vi "Configure Data Logging.vi"(7 "State (False)":bool, 8 "error in (no error)":errorcluster, 9 "Duration (30 minutes)":i32=30, 10 "Source (0:Channel 1)":i32(ring) items=["Channel 1", "Channel 2", "Channel 3", "Channel 4", "Math", "FFT"], 11 "VISA resource name":refnum<visa-resource-name>) -> (0 "error out":errorcluster, 3 "VISA resource name out":refnum<visa-resource-name>)   [LabVIEW 2015, in "Tektronix TDS 200 1000 2000 Series.lvlib"]
doc: "This VI configures the settings for the data logging."
uses:
  <instrlib>/Tektronix TDS 200 1000 2000 Series/Tektronix TDS 200 1000 2000 Series.lvlib
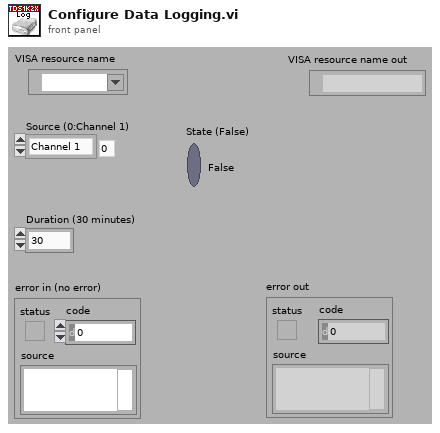
[diagram p1: front panel]
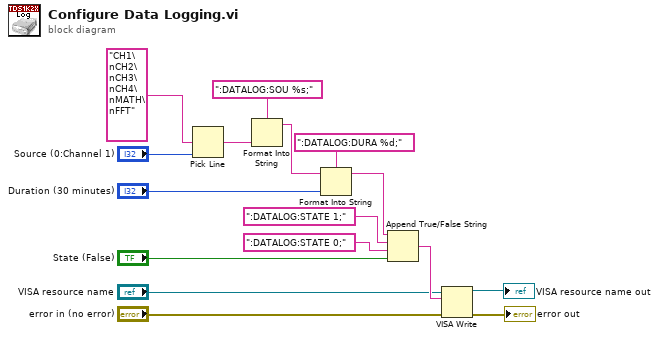
[diagram p0: block diagram]
diagram:
  n1 = Pick Line(multi-line string="CH1\nCH2\nCH3\nCH4\nMATH\nFFT", line index="Source (0:Channel 1)") -> (output string=w11:string)  [unwired: 1 out]
  n2 = Format Into String(format string=":DATALOG:SOU %s;", w11) -> (resulting string=w8:string)  [unwired: 2 in, 1 out]
  n3 = Format Into String(format string=":DATALOG:DURA %d;", initial string=w8, "Duration (30 minutes)") -> (resulting string=w7:string)  [unwired: 1 in, 1 out]
  n4 = Append True/False String(1:"State (False)", 2:":DATALOG:STATE 0;", 3:":DATALOG:STATE 1;", 4:w7) -> (0:w9:string)
  n5 = VISA Write(VISA resource name="VISA resource name", write buffer=w9, error in (no error)="error in (no error)") -> (VISA resource name out=→"VISA resource name out":refnum<visa-resource-name>, error out=→"error out":errorcluster)  [unwired: 1 out]
